vi "IPS Set Switch Heater.vi"(4 "Error In":errorcluster, 6 "Switch Heater":T1, 7 "VISA resource name":refnum<visa-resource-name>="GPIB0::24::INSTR") -> (0 "Error Out":errorcluster, 2 "Response":string="H\r", 3 "VISA resource name":refnum<visa-resource-name>="GPIB1::25::INSTR")   [LabVIEW 2016, in "IPS-120.lvlib"]
uses:
  IPS-120.lvlib
  Typedefs/Set Switch Heater - Enum.ctl
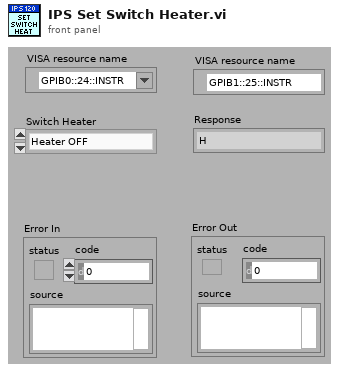
[diagram p1: front panel]
types:
  T1 = typedef "IPS-120.lvlib/Set Switch Heater - Enum.ctl" = enum16{"Heater OFF", "Heater ON if PSU=Magnet", "Heater ON, No Checks"}
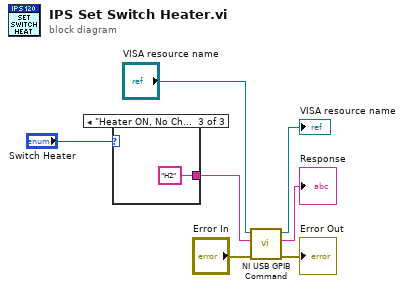
[diagram p0: block diagram]
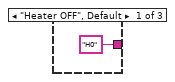
[diagram p2: hidden frame]
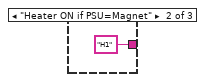
[diagram p3: hidden frame]
diagram:
  n1 = case shown="\"Heater ON, No Checks\"" "Switch Heater" {
    tunnel: ["H0" "H1" "H2"] -> w3
    frame "Heater OFF", Default {
    }
    frame "Heater ON if PSU=Magnet" {
    }
    frame "Heater ON, No Checks" {
    }
  }
  n2 = call "NI USB GPIB Command.vi"("Error In"="Error In", "write buffer"=w3, "VISA resource name"="VISA resource name") -> ("Error Out"=→"Error Out":errorcluster, "read buffer"=→"Response":string, "VISA resource name out"=→"VISA resource name":refnum<visa-resource-name>)  [unwired: 6 in]
